vi "Remove Vi.vi"(7 "Maitiain Vivalue(F)":bool=TRUE, 8 "error in":errorcluster caption="错误输入（无错误）", 9 "Abort VI":bool, 11 "PanelDataNode 输入":refnum<class "PanelDataNode.lvclass"> caption="DNL_LabVIEW Object in") -> (0 "error out":errorcluster caption="错误输出", 1 "VI*":refnum<vi>, 2 "ViValue":string, 3 "PanelDataNode 输出":refnum<class "PanelDataNode.lvclass"> caption="DNL_LabVIEW Object out")   [LabVIEW 2016, in "PanelDataNode.lvclass"]
uses:
  PanelDataNode.lvclass
  PanelDataNode.lvclass/PanelDataNode.ctl
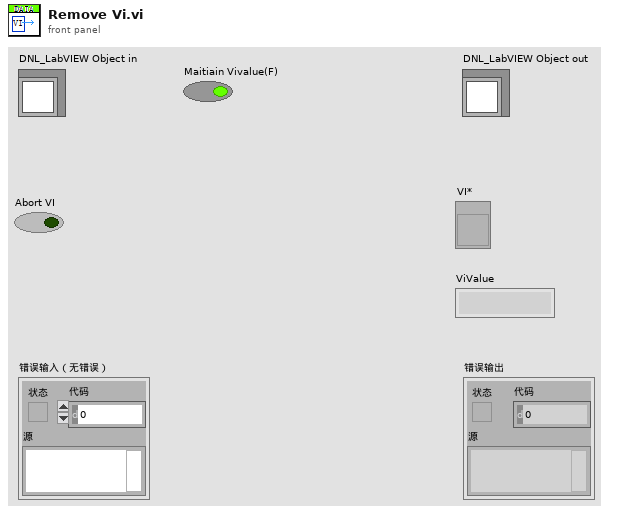
[diagram p1: front panel]
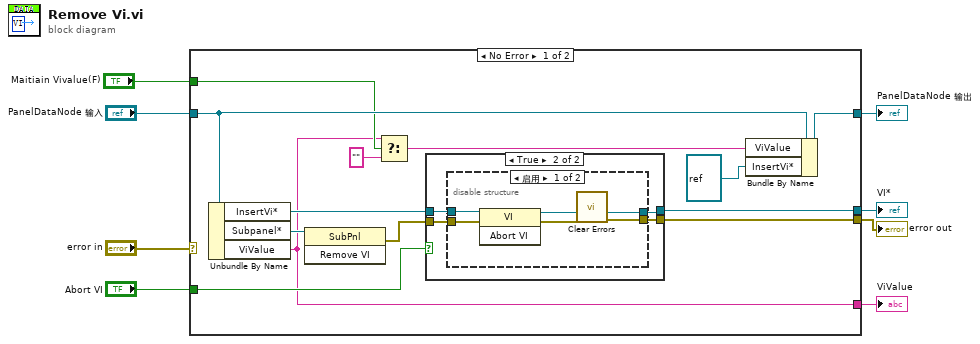
[diagram p0: block diagram]
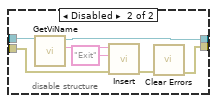
[diagram p3: hidden frame]
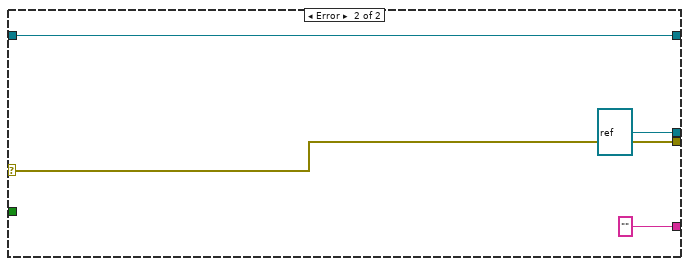
[diagram p4: hidden frame]
diagram:
  n1 = case shown="No Error" "error in" {
    selector: "error in" -> [_ w43]
    tunnel: [w13 w43] -> w7
    tunnel: [w16 w42] -> w5
    tunnel: "PanelDataNode 输入" -> [w17 w42]
    tunnel: [w18 refnum<vi> refnum ("VI*")] -> w4
    tunnel: "Abort VI" -> [w19 _]
    tunnel: [w10 "" ("ViValue")] -> w2
    tunnel: "Maitiain Vivalue(F)" -> [w12 _]
    frame No Error {
      n2 = Unbundle By Name(w17) -> ("InsertVi*"=w20:refnum<vi>, "Subpanel*"=w21:refnum<vi>, "ViValue"=w10:string)
      n3 = invoke class="SubPnl" method="Remove VI"(reference=w21) -> (error out=w14:errorcluster)  [unwired: 2 in, 2 out]
      n4 = Select(t=w10, s=w12, f="") -> (s? t:f=w11:string)
      n5 = case shown="True" w19 {
        tunnel: w20 -> [w23 w25]
        tunnel: [w23 w27] -> w18
        tunnel: [w22 w26] -> w13
        tunnel: w14 -> [w22 w24]
        frame False {
        }
        frame True {
          n6 = disable-structure shown="启用" {
            disable-tunnel: [w32 w35] -> w27
            disable-tunnel: [w30 w34] -> w26
            disable-tunnel: w25 -> [w29 w39]
            disable-tunnel: w24 -> [w28 w36]
            frame Enabled {
              n7 = invoke class="VI" method="Abort VI"(reference=w29, error in=w28) -> (reference out=w32:refnum<vi>, error out=w31:errorcluster)  [unwired: 1 in, 1 out]
              n8 = call <vilib>:"Clear Errors.vi"("error in (no error)"=w31) -> ("error out"=w30:errorcluster)  [unwired: 5 in, 1 out]
            }
            frame Disabled {
              n9 = call "GetViName.vi"("VI*"=w39) -> ("VI Name"=w38:string, "VI* out"=w35:refnum<vi>)  [unwired: 9 in]
              n10 = call "Insert.vi"("error in"=w36, "Event"="Exit", "QueueName"=w38) -> ("error out"=w33:errorcluster)  [unwired: 7 in, 1 out]
              n11 = call <vilib>:"Clear Errors.vi"("error in (no error)"=w33) -> ("error out"=w34:errorcluster)  [unwired: 5 in, 1 out]
            }
          }
        }
      }
      n12 = Bundle By Name(cluster=w17, "ViValue"=w11, "InsertVi*"=refnum<vi> refnum ("VI*")) -> (w16:refnum<class "PanelDataNode.lvclass">)
    }
    frame Error {
    }
  }
  "error out" <- w7
  "PanelDataNode 输出" <- w5
  "VI*" <- w4
  "ViValue" <- w2
